vi "Limit Array.vi"(8 "Inclination Angle In":dbl[](array[numeric]), 11 "Timestamp In":dbl[](array[numeric])) -> (0 "Inclination Angle Out":dbl[](array[numeric]), 3 "Timestamp Out":dbl[](array[numeric]))   [LabVIEW 2016, in "M1M3SupportEUI_Views.lvlib"]
uses:
  M1M3SupportEUI_Views.lvlib
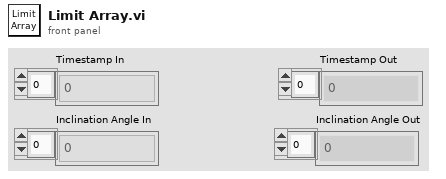
[diagram p1: front panel]
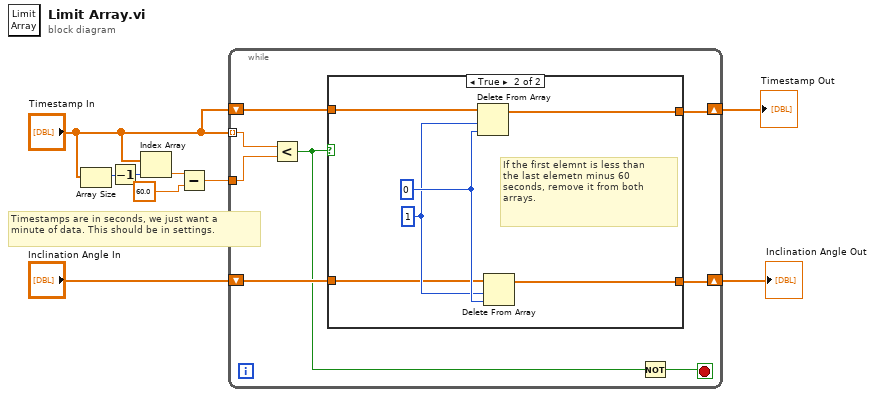
[diagram p0: block diagram]
diagram:
  # "Timestamps are in seconds, we just want a\nminute of data. This should be in settings."
  n1 = Array Size(array="Timestamp In") -> (size(s)=w7:i32)
  n2 = Decrement(x=w7) -> (x-1=w8:i32)
  n3 = Index Array(array="Timestamp In", index=w8) -> (element=w6:dbl)
  n4 = Subtract(x=w6, y=60.0) -> (x-y=w4:dbl)
  n5 = while {
    tunnel: "Timestamp In" -> [w17] mode=indexing
    tunnel: w4 -> [w16]
    shift-right: [w13] -> w2
    shift-left: "Timestamp In" -> [w15]
    shift-right: [w12] -> w1
    shift-left: "Inclination Angle In" -> [w14]
    stop <- w10 stop-if-true
    n6 = Less?(x=w17, y=w16) -> (x < y?=w11:bool)
    n7 = case shown="True" w11 {
      tunnel: w15 -> [w19 w21]
      tunnel: w14 -> [w18 w23]
      tunnel: [w18 w22] -> w12
      tunnel: [w19 w20] -> w13
      frame False {
      }
      frame True {
        w24 = 1
        w25 = 0
        # "If the first elemnt is less than\nthe last elemetn minus 60 \nseconds, remove it from both\narrays."
        n8 = Delete From Array(array=w21, length=w24, index=w25) -> (array with subset deleted=w20:dbl[])  [unwired: 1 out]
        n9 = Delete From Array(array=w23, length=w24, index=w25) -> (array with subset deleted=w22:dbl[])  [unwired: 1 out]
      }
    }
    n10 = Not(x=w11) -> (.not. x?=w10:bool)
  }
  "Timestamp Out" <- w2
  "Inclination Angle Out" <- w1
